vi "SRV_PM_VIG_WIP Byte Array Size.vi"(6 "Method (Get)":enum16{"Get", "Set"}(ring), 8 "error in (no error)":errorcluster, 10 "WIP Size":i32) -> (0 "error out":errorcluster, 2 "WIP Size out":i32)   [LabVIEW 2014]
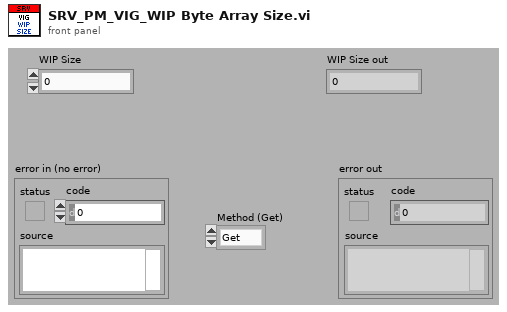
[diagram p1: front panel]
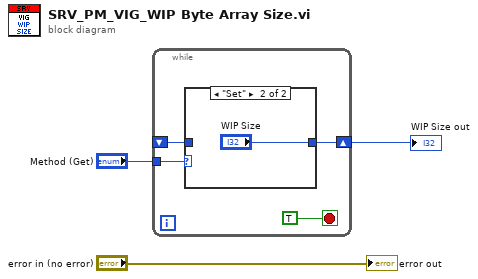
[diagram p0: block diagram]
diagram:
  n1 = while {
    tunnel: "Method (Get)" -> [w7]
    shift-right: [w5] -> w1
    shift-left: _ -> [w6]
    stop <- TRUE stop-if-true
    n2 = case shown="\"Set\"" w7 {
      tunnel: w6 -> [w8 _]
      tunnel: [w8 "WIP Size"] -> w5
      frame "Get" {
      }
      frame "Set" {
      }
    }
  }
  "WIP Size out" <- w1
  "error out" <- "error in (no error)"
